vi "VeriStand DSF.Transfer Group.Configuration.Verify.Contiguous Engine Offsets.vi"(8 "error in (no error)":errorcluster, 11 "Transfer Group Configuration in":refnum<class "VeriStand DSF.Transfer Group.Configuration.lvclass">) -> (0 "error out":errorcluster, 3 "Transfer Group Configuration out":refnum<class "VeriStand DSF.Transfer Group.Configuration.lvclass">)   [LabVIEW 2017, in "Data Sharing Framework Engine.lvlib" / "VeriStand DSF.Transfer Group.Configuration.lvclass"]
uses:
  VeriStand DSF.Transfer Group.Configuration.lvclass
  DSF Core/Built/Windows/Engine/DSF.Engine.lvlibp/DSF Configuration API/1.0.0/Public/Controls/DSF Data Type.ctl
  DSF Core/Built/Windows/Engine/DSF.Engine.lvlibp/Shared/Classes/Transfer Group/DSF.Shared.Configuration.Transfer Group.lvclass
  DSF Core/Built/Windows/Engine/DSF.Engine.lvlibp/Shared/Classes/Transfer/DSF.Shared.Configuration.Transfer.lvclass
  DSF Core/Built/Windows/Engine/DSF.Engine.lvlibp/DSF Configuration API/1.0.0/DSF Configuration API.lvlib
  DSF Core/Built/Windows/Engine/DSF.Engine.lvlibp
  C:/Git/DSF/DSF Core/Built/Windows/Engine/DSF.Engine.lvlibp/Shared/Classes/Transfer Group/DSF.Shared.Configuration.Transfer Group.lvclass
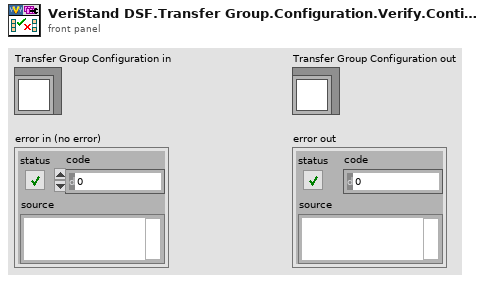
[diagram p1: front panel]
types:
  T1 = typedef "DSF.Engine.lvlibp/DSF Configuration API.lvlib/DSF Data Type.ctl" = enum8{"Bool", "SGL", "DBL", "I8", "I16", "I32", "I64", "U8", "U16", "U32", "U64"}
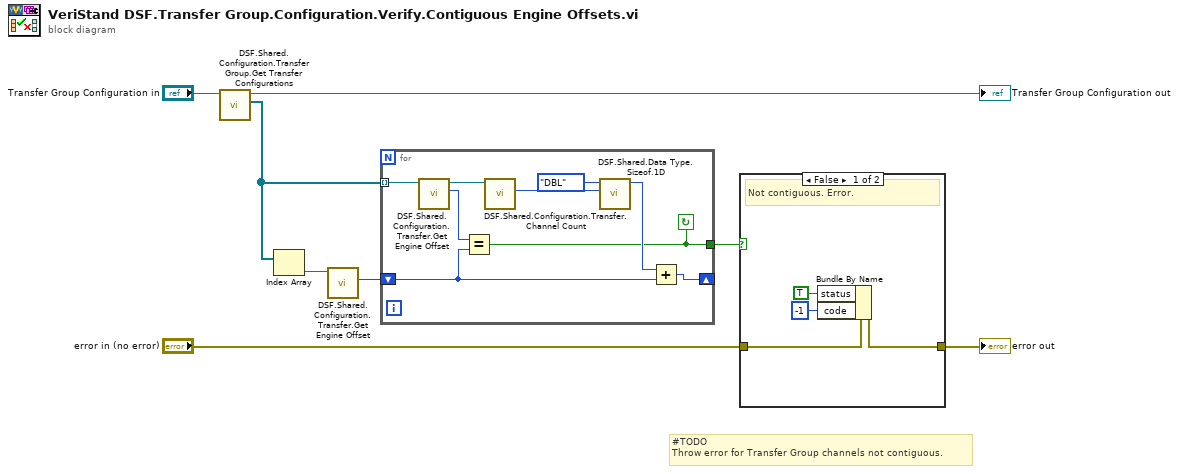
[diagram p0: block diagram]
diagram:
  # "#TODO\nThrow error for Transfer Group channels not contiguous."
  n1 = call "DSF.Shared.Configuration.Transfer Group.Get Transfer Configurations.vi"("Transfer Group Configuration in"="Transfer Group Configuration in") -> ("Transfer Configurations"=w5:refnum<class "DSF.Shared.Configuration.Transfer.lvclass">[], "Transfer Group Configuration out"=→"Transfer Group Configuration out":refnum<class "VeriStand DSF.Transfer Group.Configuration.lvclass">)  [unwired: 9 in]
  n2 = Index Array(array=w5) -> (element=w3:refnum<class "DSF.Shared.Configuration.Transfer.lvclass">)  [unwired: 1 in]
  n3 = call "DSF.Shared.Configuration.Transfer.Get Engine Offset.vi"("Transfer Configuration in"=w3) -> ("engine offset"=w4:u64)  [unwired: 9 in, 1 out]
  n4 = for {
    shift-right: [w10] -> _
    shift-left: w4 -> [w14]
    tunnel: w5 -> [w17] mode=indexing
    tunnel: [w9] -> w8
    stop <- w9 continue-if-true
    n5 = call "DSF.Shared.Configuration.Transfer.Get Engine Offset.vi"("Transfer Configuration in"=w17) -> ("engine offset"=w15:u64, "Transfer Configuration out"=w16:refnum<class "DSF.Shared.Configuration.Transfer.lvclass">)  [unwired: 9 in]
    n6 = Equal?(x=w15, y=w14) -> (x = y?=w9:bool)
    n7 = call "DSF.Shared.Configuration.Transfer.Channel Count.vi"("Transfer Configuration in"=w16) -> ("total channel count"=w12:u64)  [unwired: 8 in, 2 out]
    n8 = call "DSF.Shared.Data Type.Sizeof.1D.vi"("count"=w12, "data type"=DSF_Data_Type."DBL") -> ("size in bytes"=w11:u64)  [unwired: 9 in]
    n9 = Add(x=w11, y=w14) -> (x+y=w10:u64)
  }
  n10 = case shown="False" w8 {
    tunnel: "error in (no error)" -> [w21 w22]
    tunnel: [w20 w22] -> w7
    frame False {
      # "Not contiguous. Error."
      n11 = Bundle By Name(cluster=w21, "status"=TRUE, "code"=-1) -> (w20:errorcluster)
    }
    frame True {
      # "Contiguous. Proceed."
    }
  }
  "error out" <- w7
